vi "Target Phase Calculator.vi"(8 "Count":i32, 11 "HS Detected":bool) -> (3 "Phase":dbl)   [LabVIEW 2018, in "COBRA Gait Phase Estimation Library.lvlib"]
uses:
  COBRA Gait Phase Estimation Library.lvlib
  <vilib>/ptbypt/NI_PtbyPt.lvlib
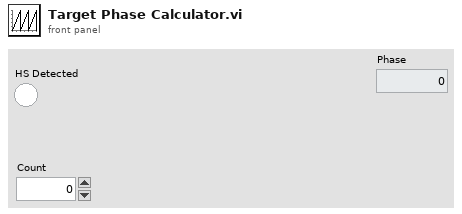
[diagram p1: front panel]
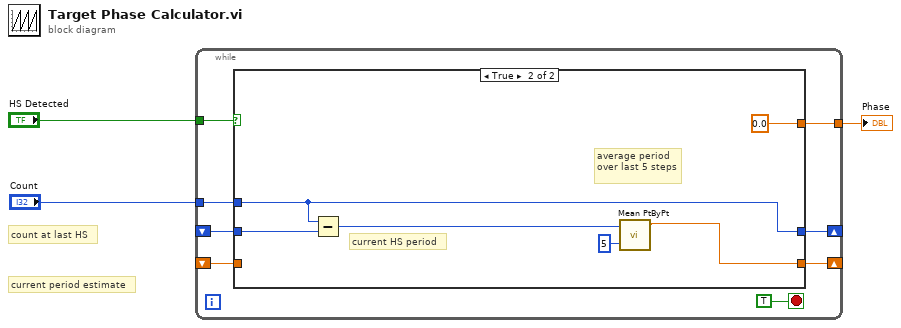
[diagram p0: block diagram]
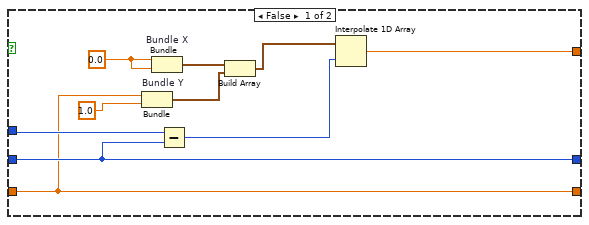
[diagram p2: hidden frame]
diagram:
  # "current period estimate"
  # "count at last HS"
  n1 = while {
    tunnel: "HS Detected" -> [w10]
    tunnel: [w9] -> w2
    tunnel: "Count" -> [w8]
    shift-right: [w5] -> _
    shift-left: _ -> [w7]
    shift-right: [w6] -> _
    shift-left: _ -> [w4]
    stop <- TRUE stop-if-true
    n2 = case shown="True" w10 {
      tunnel: [w19 0.0] -> w9
      tunnel: w8 -> [w21 w26]
      tunnel: [w20 w26] -> w5
      tunnel: w7 -> [w20 w25]
      tunnel: [w15 w23] -> w6
      tunnel: w4 -> [w15 _]
      frame False {
        w18 = 0.0
        n3 = Bundle "Bundle Y"("mean"=w15, 1.0) -> (w14:cluster{"mean":dbl, dbl})  [unwired: 1 in]
        n4 = Bundle "Bundle X"(w18, w18) -> (w17:cluster{dbl, dbl})  [unwired: 1 in]
        n5 = Subtract(x=w21, y=w20) -> (x-y=w12:i32)
        n6 = Build Array "Build Array"(w17, w14) -> (w13:cluster{"mean":dbl, dbl}[])
        n7 = Interpolate 1D Array(1:w12, 2:w13) -> (0:w19:dbl)
      }
      frame True {
        # "average period\nover last 5 steps"
        # "current HS period"
        n8 = Subtract(x=w26, y=w25) -> (x-y=w24:i32)
        n9 = call <vilib>:"Mean PtByPt.vi"("x"=w24, "sample length"=5) -> ("mean"=w23:dbl)  [unwired: 2 in, 1 out]
      }
    }
  }
  "Phase" <- w2
